vi "ReadINI.vi"(11 "error in":errorcluster) -> (4 "Button":T1, 8 "Found?":bool, 15 "error out":errorcluster)   [LabVIEW 2020]
uses:
  ButtonDialogEnum.ctl
  <vilib>/Utility/config.llb/Read Key (String).vi
  <vilib>/Utility/config.llb/NI_LVConfig.lvlib
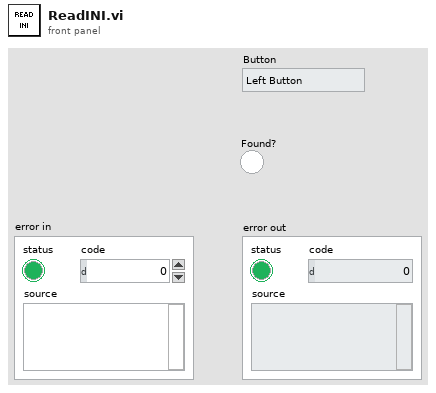
[diagram p1: front panel]
types:
  T1 = typedef "ButtonDialogEnum.ctl" = enum16{"Left Button", "Middle Button", "Right Button", "Window Close"}
  T2 = typedef "NI_LVConfig.lvlib/Config Data RefNum.ctl" = refnum<k1>
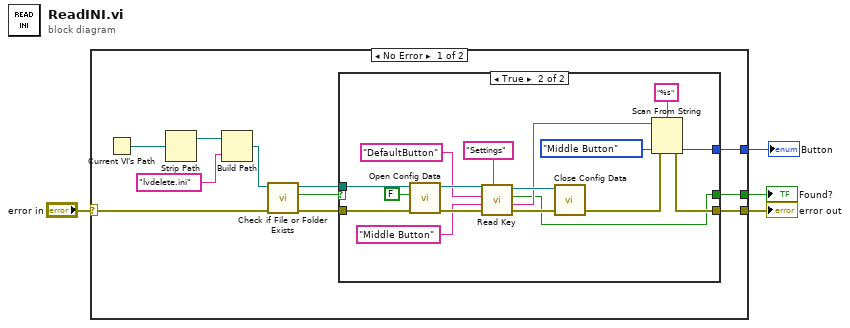
[diagram p0: block diagram]
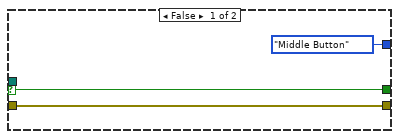
[diagram p2: hidden frame]
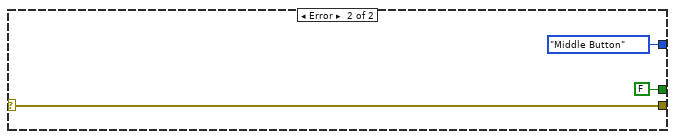
[diagram p3: hidden frame]
diagram:
  n1 = case shown="No Error" "error in" {
    selector: "error in" -> [w7 w38]
    tunnel: [w8 w38] -> w4
    tunnel: [w6 FALSE ("found?")] -> w2
    tunnel: [w5 ButtonDialogEnum."Middle Button" ("Enum")] -> w1
    frame No Error {
      n2 = Current VI's Path() -> (path=w15:path)
      n3 = Strip Path(path=w15) -> (stripped path=w14:path)  [unwired: 1 out]
      n4 = Build Path(base path=w14, name or relative path="lvdelete.ini") -> (appended path=w12:path)
      n5 = call <vilib>:"Check if File or Folder Exists.vi"("error in (no error)"=w7, "path"=w12) -> ("error out"=w9:errorcluster, "file or folder exists?"=w11:bool, "dup path"=w10:path)  [unwired: 7 in]
      n6 = case shown="True" w11 {
        selector: w11 -> [w17 _]
        tunnel: w10 -> [_ w35]
        tunnel: w9 -> [w18 w33]
        tunnel: [w18 w21] -> w8
        tunnel: [w17 w20] -> w6
        tunnel: [ButtonDialogEnum."Middle Button" ("Enum") w19] -> w5
        frame False {
        }
        frame True {
          n7 = call <vilib>:"Open Config Data.vi"("error in (no error)"=w33, "create file if necessary (T)"=FALSE, "configuration file path"=w35) -> ("error out"=w31:errorcluster, "refnum"=w32:T2)  [unwired: 6 in, 1 out]
          n8 = call-poly <vilib>:"Read Key.vi"("section"="Settings", "error in (no error)"=w31, "default value"="Middle Button", "key"="DefaultButton", "refnum"=w32) -> ("error out"=w29:errorcluster, "value"=w24:string, "found?"=w20:bool, "refnum out"=w30:T2)  [unwired: 3 in]
          n9 = call <vilib>:"Close Config Data.vi"("error in (no error)"=w29, "refnum"=w30) -> ("error out"=w22:errorcluster)  [unwired: 8 in, 1 out]
          n10 = Scan From String(format string="%s", input string=w24, error in=w22, default 1=ButtonDialogEnum."Middle Button" ("Enum")) -> (error out=w21:errorcluster, output 1=w19:T1)  [unwired: 1 in, 2 out]
        }
      }
    }
    frame Error {
    }
  }
  "error out" <- w4
  "Found?" <- w2
  "Button" <- w1
